vi "Indexer.vi"(8 "error in (no error)":errorcluster, 11 "Robot Commands":T1) -> (0 "error out":errorcluster)   [LabVIEW 2014]
uses:
  SubSystems/Robot Commands.ctl
  <vilib>/Rock Robotics/WPI/Relay/WPI_RelayValue.ctl
  Global Variables/Global Variables.vi
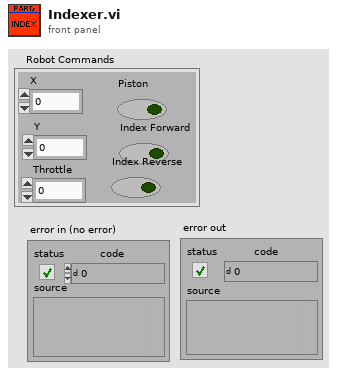
[diagram p1: front panel]
types:
  T1 = typedef "Robot Commands.ctl" = cluster{"X":dbl, "Y ":dbl, "Throttle":dbl, "Piston":bool, "Index Forward":bool, "Index Reverse ":bool}
  T2 = typedef "WPI_RelayValue.ctl" = enum16{"Off", "On", "Forward", "Reverse"}
  T3 = typedef "WPI_RelayDevRef.ctl" = cluster{"DevStatus":errorcluster, "Relay Channel":T4, "Controller":T5, "Relay Direction":T6}
  T4 = typedef "FPGA_DIORelayChannel.ctl" = enum8{"Relay 0", "Relay 1", "Relay 2", "Relay 3", "Invalid"}
  T5 = typedef "FPGA_TypedefDigitalModule.ctl" = enum16{"Controller 1"}
  T6 = typedef "WPI_RelayDirection.ctl" = enum16{"Both directions", "Forward only", "Reverse only"}
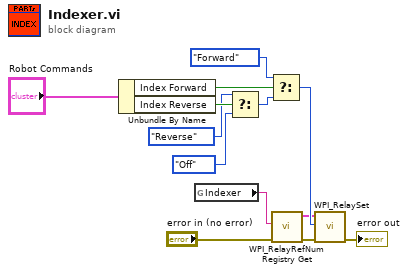
[diagram p0: block diagram]
diagram:
  n1 = Unbundle By Name("Robot Commands") -> ("Index Forward"=w12:bool, "Index Reverse"=w10:bool)
  n2 = global read "Global Variables.vi" "Indexer"() -> (w3:string)
  n3 = Select(t=WPI_RelayValue."Reverse" ("RelayValue"), s=w10, f=WPI_RelayValue."Off" ("RelayValue")) -> (s? t:f=w8:T2)
  n4 = Select(t=WPI_RelayValue."Forward" ("RelayValue"), s=w12, f=w8) -> (s? t:f=w7:T2)
  n5 = call <vilib>:"WPI_RelayRefNum Registry Get.vi"("error in (no error)"="error in (no error)", "refnum name"=w3) -> ("error out"=w5:errorcluster, "RelayDevRef"=w4:T3)  [unwired: 8 in]
  n6 = call <vilib>:"WPI_RelaySet.vi"("error in (no error)"=w5, "RelayValue"=w7, "RelayDevRef"=w4) -> ("error out"=→"error out":errorcluster)  [unwired: 7 in, 1 out]
